vi "Write Columns.vi"(8 "error in (no error)":errorcluster, 10 "Columns":T1(c390), 11 "Basic Table in":refnum<class "Basic Table.lvclass">) -> (0 "error out":errorcluster, 3 "Basic Table out":refnum<class "Basic Table.lvclass">)   [LabVIEW 2020, in "Table.lvlib" / "Basic Table.lvclass"]
uses:
  Basic Table.lvclass
  Column Libraries/Column Interface/Column Interface Class/Column Interface.lvclass
  Basic Table.lvclass/Basic Table.ctl
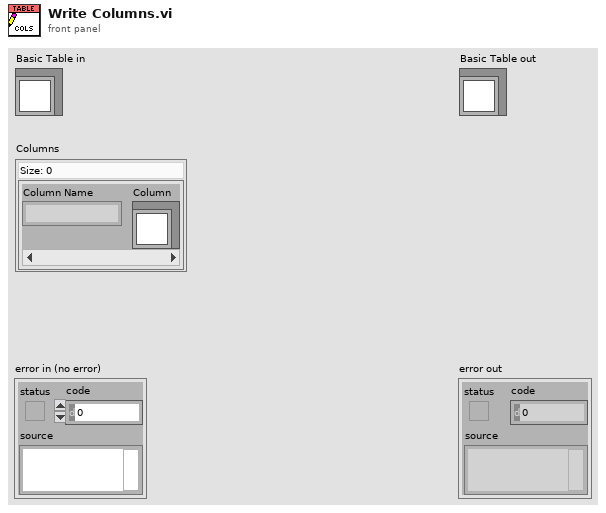
[diagram p1: front panel]
types:
  T1 = map{string, refnum<class "Column Interface.lvclass">}
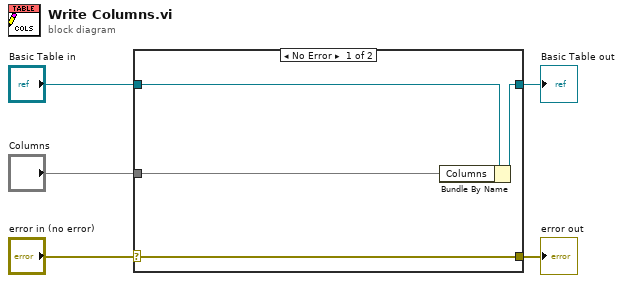
[diagram p0: block diagram]
diagram:
  n1 = case shown="No Error" "error in (no error)" {
    selector: "error in (no error)" -> [w9 w10]
    tunnel: [w9 w10] -> w4
    tunnel: [w7 w11] -> w2
    tunnel: "Basic Table in" -> [w8 w11]
    tunnel: "Columns" -> [w6 _]
    frame No Error {
      n2 = Bundle By Name(cluster=w8, "Columns"=w6) -> (w7:refnum<class "Basic Table.lvclass">)
    }
    frame Error {
    }
  }
  "error out" <- w4
  "Basic Table out" <- w2
